vi "Test Stopwatch.vi"(11 "Error in":errorcluster) -> (15 "Error out":errorcluster)   [LabVIEW 2020, in "StopWatchTests.lvlib"]
doc: "This VI is used for validating stopwatch"
uses:
  StopWatchTests.lvlib
  <vilib>/SLL Drona/APIs/Stimulus/ControlValue/SetValueAuto.vi
  <vilib>/SLL Drona/APIs/Assert/AssertControlValue/AlmostEqual.vi
  <vilib>/SLL Drona/APIs/Assert/AssertControlValue/Equal.vi
  <vilib>/SLL Drona/APIs/Stimulus/VI/CloseVI.vi
  <vilib>/addons/_JKI Toolkits/Caraya/classes/Test/Test.lvclass
  <vilib>/SLL Drona/Drona.lvlib
  <vilib>/SLL Drona/APIs/Stimulus/ControlValue/ControlValue.lvlib
  <vilib>/SLL Drona/APIs/Assert/AssertControlValue/AssertControlValue.lvlib
  <vilib>/SLL Drona/APIs/Stimulus/VI/VI.lvlib
panel:
  # "STOPWATCH TEST"
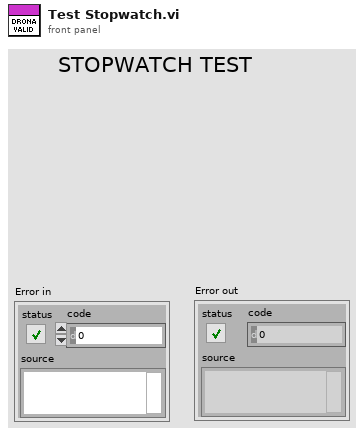
[diagram p1: front panel]
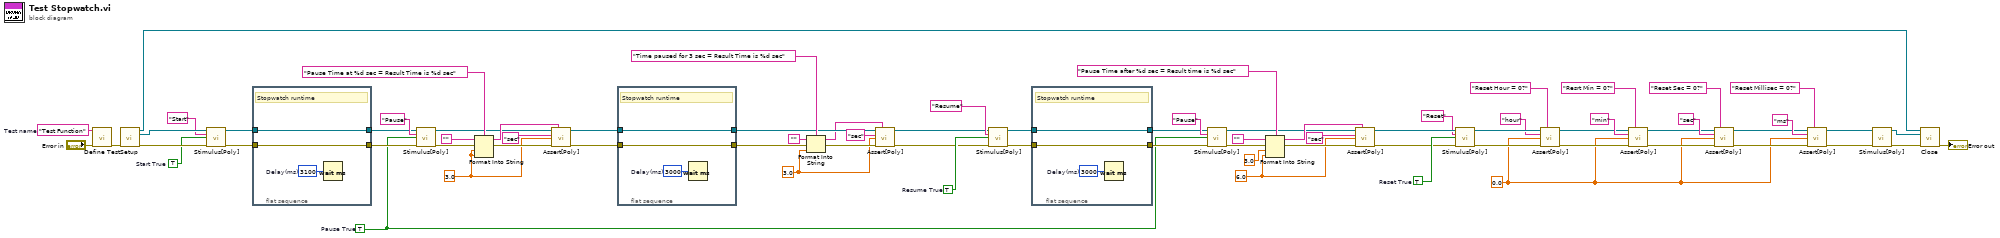
[diagram p0: block diagram]
diagram:
  w6 = 3.0 ("input 1")
  w20 = 0.0 ("input 1")
  w41 = TRUE  # Reset True
  w43 = 6.0 ("input 1")
  w56 = TRUE  # Resume True
  w44 = 3.0 ("input 1")
  w38 = TRUE  # Pause True
  w68 = TRUE  # Start True
  w75 = "Test Function"  # Test name
  n1 = call <vilib>:"Define Test.vi"("error in (no error)"="Error in", "Label (VI Title)"=w75) -> ("error out"=w74:errorcluster)  [unwired: 9 in]
  n2 = call <vilib>:"Setup.vi"("error in"=w74) -> ("Application Ref"=w70:refnum<vi>, "VI Reference Out"=w72:refnum<vi>, "error out"=w73:errorcluster)  [unwired: 12 in]
  n3 = call-poly <vilib>:"Stimulus[Poly].vi"("VI Reference In"=w72, "Control Path"="Start", "Value (Signaling)"=w68, "error in"=w73) -> ("VI Reference Out"=w63:refnum<vi>, "error out"=w67:errorcluster)  [unwired: 10 in]
  n4 = flat-sequence {
    tunnel: w67 -> [w79]
    tunnel: [w79] -> w66
    tunnel: [w77] -> w64
    tunnel: w63 -> [w77]
    frame #0 {
      w78 = u32 3100  # Delay(ms)
      # "Stopwatch runtime"
      n5 = Wait (ms)(milliseconds to wait=w78) -> ()  [unwired: 1 out]
    }
  }
  n6 = call-poly <vilib>:"Stimulus[Poly].vi"("VI Reference In"=w64, "Control Path"="Pause", "Value (Signaling)"=w38, "error in"=w66) -> ("VI Reference Out"=w18:refnum<vi>, "error out"=w62:errorcluster)  [unwired: 10 in]
  n7 = Format Into String(format string="Pause Time at %d sec = Result Time is %d sec", initial string="", error in=w62, w44, w44) -> (resulting string=w59:string, error out=w61:errorcluster)
  n8 = call-poly <vilib>:"Assert[Poly].vi"("VI Reference In"=w18, "Test Label"=w59, "Control Path"="sec", "Control Value"=w44, "Error In"=w61) -> ("VI Reference Out"=w17:refnum<vi>, "Error Out"=w16:errorcluster)  [unwired: 9 in]
  n9 = flat-sequence {
    tunnel: w16 -> [w82]
    tunnel: [w82] -> w15
    tunnel: [w80] -> w11
    tunnel: w17 -> [w80]
    frame #0 {
      w81 = u32 3000  # Delay(ms)
      # "Stopwatch runtime"
      n10 = Wait (ms)(milliseconds to wait=w81) -> ()  [unwired: 1 out]
    }
  }
  n11 = Format Into String(format string="Time paused for 3 sec = Result Time is %d sec", initial string="", error in=w15, w6) -> (resulting string=w8:string, error out=w12:errorcluster)
  n12 = call-poly <vilib>:"Assert[Poly].vi"("VI Reference In"=w11, "Test Label"=w8, "Control Path"="sec", "Control Value"=w6, "Error In"=w12) -> ("VI Reference Out"=w9:refnum<vi>, "Error Out"=w10:errorcluster)  [unwired: 9 in]
  n13 = call-poly <vilib>:"Stimulus[Poly].vi"("VI Reference In"=w9, "Control Path"="Resume", "Value (Signaling)"=w56, "error in"=w10) -> ("VI Reference Out"=w54:refnum<vi>, "error out"=w55:errorcluster)  [unwired: 10 in]
  n14 = flat-sequence {
    tunnel: w55 -> [w85]
    tunnel: [w85] -> w48
    tunnel: [w83] -> w49
    tunnel: w54 -> [w83]
    frame #0 {
      w84 = u32 3000  # Delay(ms)
      # "Stopwatch runtime"
      n15 = Wait (ms)(milliseconds to wait=w84) -> ()  [unwired: 1 out]
    }
  }
  n16 = call-poly <vilib>:"Stimulus[Poly].vi"("VI Reference In"=w49, "Control Path"="Pause", "Value (Signaling)"=w38, "error in"=w48) -> ("VI Reference Out"=w42:refnum<vi>, "error out"=w51:errorcluster)  [unwired: 10 in]
  n17 = Format Into String(format string="Pause Time after %d sec = Result time is %d sec", initial string="", error in=w51, 3.0 ("input 2"), w43) -> (resulting string=w45:string, error out=w46:errorcluster)
  n18 = call-poly <vilib>:"Assert[Poly].vi"("VI Reference In"=w42, "Test Label"=w45, "Control Path"="sec", "Control Value"=w43, "Error In"=w46) -> ("VI Reference Out"=w39:refnum<vi>, "Error Out"=w40:errorcluster)  [unwired: 9 in]
  n19 = call-poly <vilib>:"Stimulus[Poly].vi"("VI Reference In"=w39, "Control Path"="Reset", "Value (Signaling)"=w41, "error in"=w40) -> ("VI Reference Out"=w34:refnum<vi>, "error out"=w36:errorcluster)  [unwired: 10 in]
  n20 = call-poly <vilib>:"Assert[Poly].vi"("VI Reference In"=w34, "Test Label"="Reset Hour = 0?" ("Label"), "Control Path"="hour", "Control Value"=w20, "Error In"=w36) -> ("VI Reference Out"=w30:refnum<vi>, "Error Out"=w29:errorcluster)  [unwired: 9 in]
  n21 = call-poly <vilib>:"Assert[Poly].vi"("VI Reference In"=w30, "Test Label"="Resrt Min = 0?" ("Label"), "Control Path"="min", "Control Value"=w20, "Error In"=w29) -> ("VI Reference Out"=w25:refnum<vi>, "Error Out"=w26:errorcluster)  [unwired: 9 in]
  n22 = call-poly <vilib>:"Assert[Poly].vi"("VI Reference In"=w25, "Test Label"="Reset Sec = 0?" ("Label"), "Control Path"="sec", "Control Value"=w20, "Error In"=w26) -> ("VI Reference Out"=w21:refnum<vi>, "Error Out"=w22:errorcluster)  [unwired: 9 in]
  n23 = call-poly <vilib>:"Assert[Poly].vi"("VI Reference In"=w21, "Test Label"="Reset Millisec = 0?" ("Label"), "Control Path"="ms", "Control Value"=w20, "Error In"=w22) -> ("VI Reference Out"=w3:refnum<vi>, "Error Out"=w4:errorcluster)  [unwired: 9 in]
  n24 = call-poly <vilib>:"Stimulus[Poly].vi"("VI Reference In"=w3, "error in"=w4) -> ("VI Reference Out"=w2:refnum<vi>, "error out"=w1:errorcluster)  [unwired: 12 in]
  n25 = call <vilib>:"Close.vi"("Application Ref"=w70, "VI Reference"=w2, "error in"=w1) -> ("error out"=→"Error out":errorcluster)  [unwired: 12 in]
